vi "Gyro Steer.vi"(9 "Target Angle":dbl, 11 "Changed?":bool) -> (3 "X out":dbl)   [LabVIEW 2014]
uses:
  Robot Global Data.vi
  <vilib>/addons/control/pid/pid.llb/PID (DBL).vi
  <vilib>/addons/control/pid/NI_PID_pid.lvlib
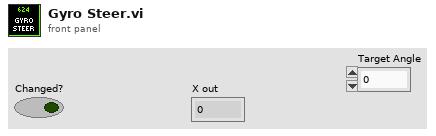
[diagram p1: front panel]
types:
  T1 = typedef "Dashboard Control Data.ctl" = cluster{"Cam Exposure":dbl, "Go to angle":dbl, "Steer PID Gains":cluster{"proportional gain (Kc)":dbl, "integral time (Ti, min)":dbl, "derivative time (Td, min)":dbl}, "Steer PID output Range":cluster{"output high":dbl, "output low":dbl}, "Pressure m \nValue":dbl, "Pressure b \nValue":dbl, "Strafe Timer\nWait":dbl, "Roller Command Cluster ":T2, "Elevator":T3, "Strafe Correct min X":dbl, "IMU Enable":bool}
  T2 = typedef "Roller Control.ctl" = cluster{"Left Roller Speed":dbl, "Right Roller Speed":dbl, "Left Roller Speed Back":dbl, "Right Roller Speed Back":dbl, "Roller Align Decide Limit":u32, "Left Roller Speed Unload":dbl, "Right Roller Speed Unload":dbl, "Ping Dist Difference":dbl}
  T3 = typedef "Elevator DB Control.ctl" = cluster{"Presets":cluster{"Hold Tote":dbl, "Hold Trashcan":dbl, "Pickup 2 w/ Tote":dbl, "Pickup 2 w/ Trashcan":dbl, "Pickup 3 w/ Tote":dbl, "Pickup 3 w/ Trashcan":dbl, "Lift Plate Deploy":dbl, "Bottom":dbl, "Lift Plate Deploy for 2":dbl, "Lift Plate Deploy for 3":dbl}, "PID Output Range":cluster{"output high":dbl, "output low":dbl}, "PID gains":cluster{"proportional gain (Kc)":dbl, "integral time (Ti, min)":dbl, "derivative time (Td, min)":dbl}, "LP Close Angle":i32, "LP Open Angle":i32, "Height Tolerance":dbl, "L Encoder Constant":dbl, "R Encoder Constant":dbl}
  T4 = cluster{"proportional gain (Kc)":dbl, "integral time (Ti, min)":dbl, "derivative time (Td, min)":dbl}
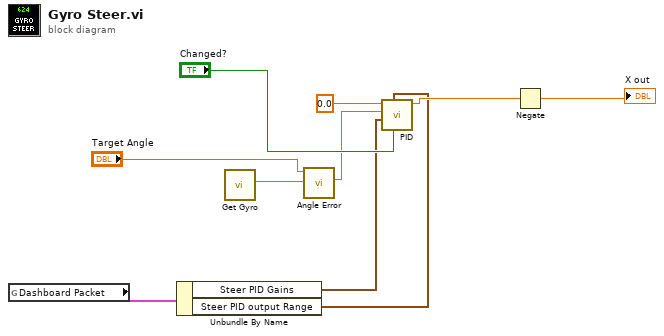
[diagram p0: block diagram]
diagram:
  n1 = global read "Robot Global Data.vi" "Dashboard Packet"() -> (w4:T1)
  n2 = Unbundle By Name(w4) -> ("Steer PID Gains"=w2:T4, "Steer PID output Range"=w1:cluster{"output high":dbl, "output low":dbl})
  n3 = call "Get Gyro.vi"() -> ("Angle"=w5:dbl)  [unwired: 11 in]
  n4 = call "Angle Error.vi"("Angle"=w5, "Target Angle"="Target Angle") -> ("Error"=w7:dbl)  [unwired: 9 in]
  n5 = call-poly <vilib>:"PID.vi"("reinitialize? (F)"="Changed?", "output range"=w1, "PID gains"=w2, "process variable"=w7, "setpoint"=0.0) -> ("output"=w8:dbl)  [unwired: 5 in, 1 out]
  n6 = Negate(x=w8) -> (-x=→"X out":dbl)
